vi "SetSerializeSliceClass.vi"(8 "error in (no error)":errorcluster, 11 "Tiger Woods in":refnum<class "Tiger Woods.lvclass">) -> (0 "error out":errorcluster, 2 "Slice-To-This Class Name":string)   [LabVIEW 2019, in "Tiger Woods.lvclass"]
uses:
  Tiger Woods.lvclass
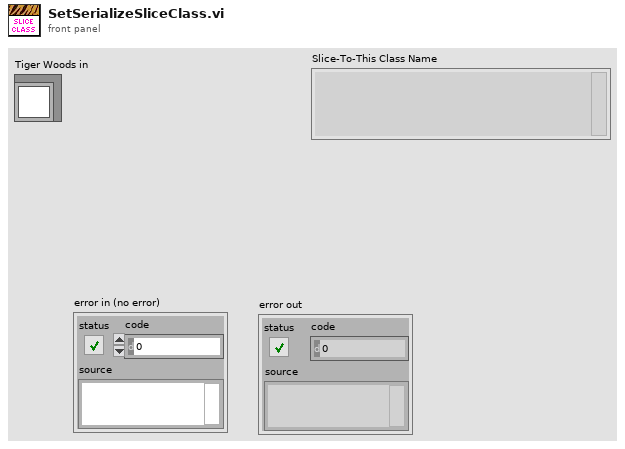
[diagram p1: front panel]
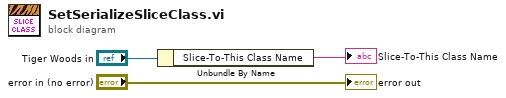
[diagram p0: block diagram]
diagram:
  n1 = Unbundle By Name("Tiger Woods in") -> ("Slice-To-This Class Name"=→"Slice-To-This Class Name":string)
  "error out" <- "error in (no error)"
